vi "Demo Multitouch.vi"(8 "error in (no error)":errorcluster) -> (0 "error out":errorcluster)   [LabVIEW 2011]
uses:
  VIremote.llb/VIremoteEvent.ctl
  VIremote.llb/VIremoteFunction.ctl
  <vilib>/Utility/miscctls.llb/LVPointTypeDef.ctl
  <vilib>/Utility/miscctls.llb/LVPositionTypeDef.ctl
  VIremote.llb/VIremoteTouchPhase.ctl
panel:
  out "VIremoteEvent":T1=enum."Connection Closed"
  out "2D Picture":picture
  # "Touch with one finger to draw.\nTouch with two fingers to draw a line between them."
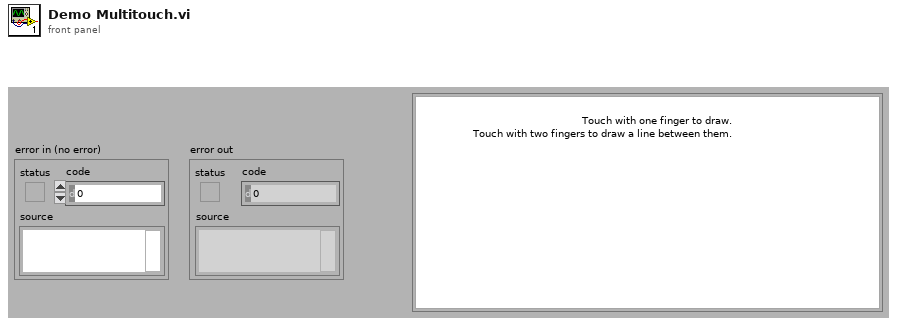
[diagram p1: front panel]
types:
  T1 = typedef "VIremoteEvent.ctl" = enum16{"No Event", "Connection Closed", "Navigate Back", "Enter Background", "Enter Foreground", "Portrait", "Portrait Upside Down", "Landscape Left", "Landscape Right"}
  T2 = typedef "LVPositionTypeDef.ctl" = cluster{"Left":i32, "Top":i32}
  T3 = typedef "LVPointTypeDef.ctl" = cluster{"Horizontal":i16, "Vertical":i16}
  T4 = typedef "VIremoteFunction.ctl" = enum16{"Do nothing", "Stop controller", "Close this connection", "Show info panel", "Set VI to control", "Set Accelerometer freq (Hz)", "Show Alert message", "Start Sound Input", "Stop Sound Input", "Set Volume (0-100)", "Set sound output Speaker", "Set sound output Receiver", "Play Sound", "Repeat Sound", "Stop Sound", "Pause Sound", "Resume Sound", "Set panel width of caller (320 or 480)", "Set Panel Size to Portrait", "Set Panel Size to Landscape", "Set Panel Size as Current Orientation", "Allow all UI Orientations", "Send user notification", "Disable Scrolling", "Normal Scrolling", "Page Scrolling", "Set Scroll Offset", "Page Indicator Position"}
  T5 = cluster{"UIorientation":refnum<notifier>, "Accelerometer":refnum<notifier>, "Sound":refnum<notifier>, "SoundPlayBufferReady":refnum<notifier>, "BackgroundState":refnum<notifier>, "Touch":refnum<notifier>}
  T6 = typedef "VIremoteTouchPhase.ctl" = enum32{"Began", "Moved", "Stationary", "Ended", "Cancelled"}
  T7 = cluster{"Width":u16, "Style":enum32{"Solid", "Dash", "Dot", "DashDot", "DashDotDot"}}
  T8 = typedef "VIremoteTouch.ctl" = cluster{"# touches":i32, "Touch phase":T6, "X":dbl, "Y":dbl, "Tap count":i32, "Timestamp":dbl, "ID":u32}
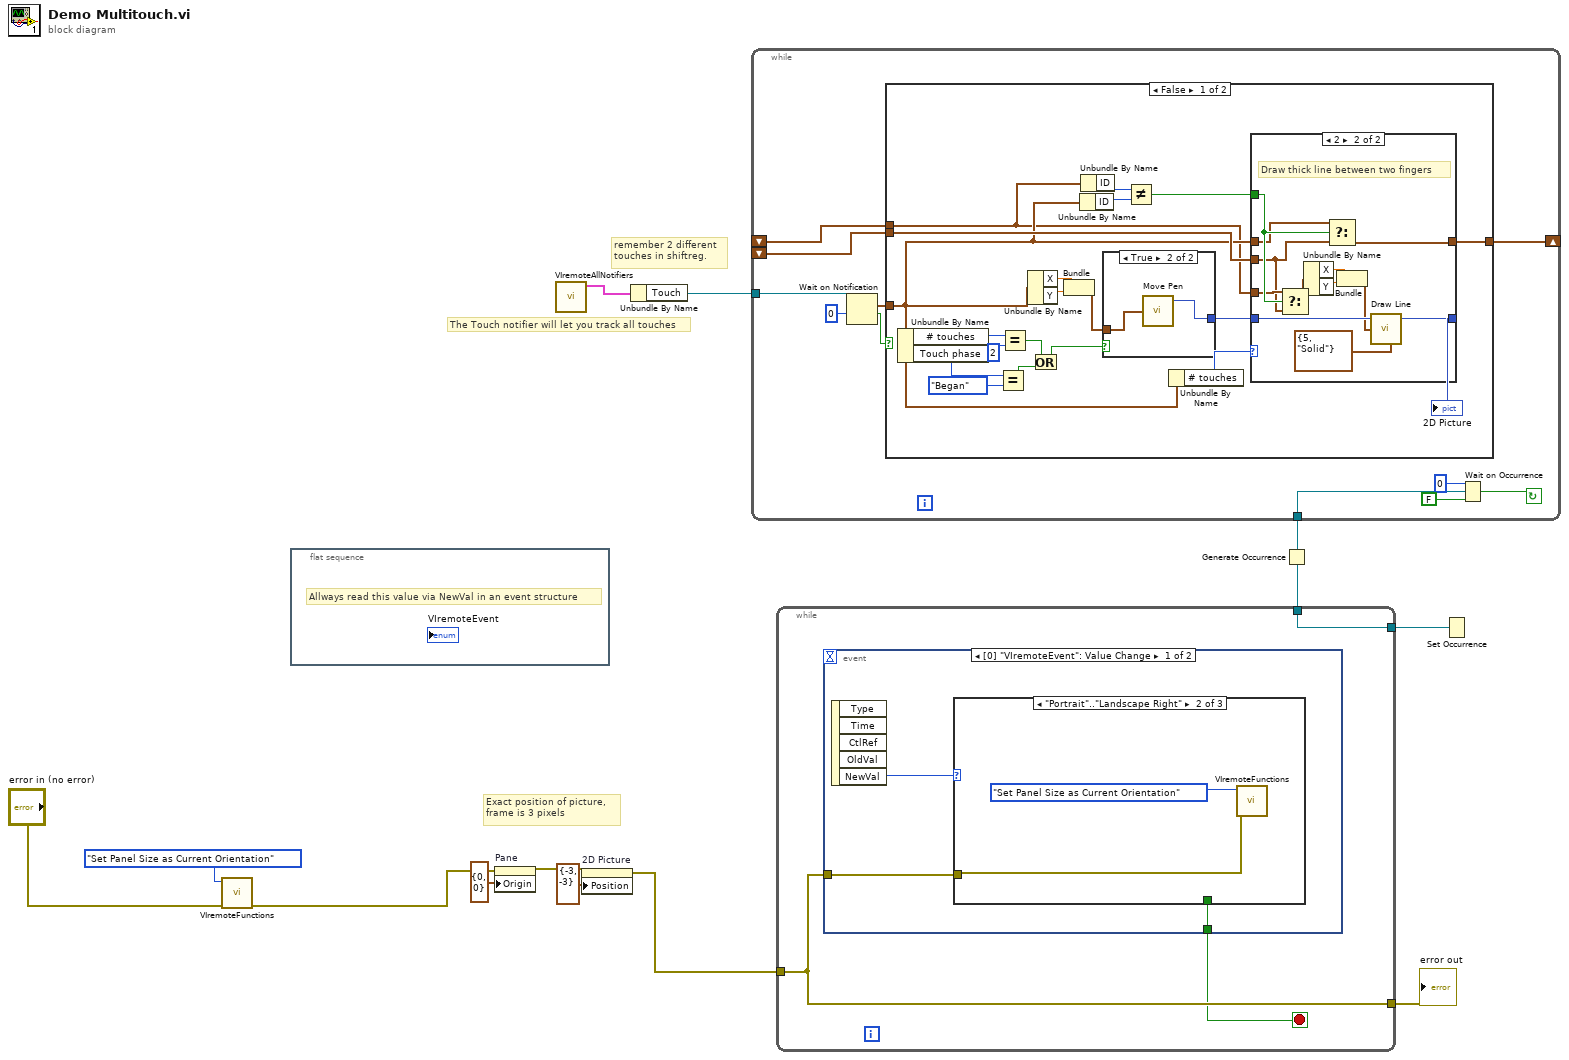
[diagram p0: block diagram]
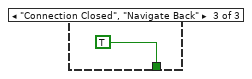
[diagram p3: hidden frame]
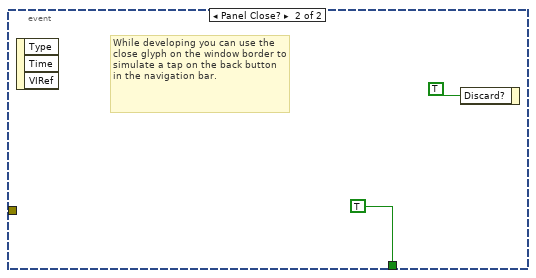
[diagram p4: hidden frame]
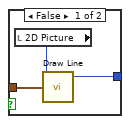
[diagram p6: hidden frame]
diagram:
  # "The Touch notifier will let you track all touches"
  # "Exact position of picture, \nframe is 3 pixels"
  # "remember 2 different\ntouches in shiftreg."
  n1 = call "VIremoteFunctions.vi"("error in (no error)"="error in (no error)", "Function"=VIremoteFunction."Set Panel Size as Current Orientation") -> ("error out"=w1:errorcluster)  [unwired: 4 in, 5 out]
  n2 = flat-sequence {
    frame #0 {
      # "Allways read this value via NewVal in an event structure"
    }
  }
  n3 = property on="Pane" class="Pane"(error in=w1, "Origin"=T3 {"Horizontal"=0, "Vertical"=0}) -> (error out=w6:errorcluster)  [unwired: 1 in, 1 out]
  n4 = call "VIremoteAllNotifiers.vi"() -> ("All Notifiers (unbundle by name)"=w11:T5)  [unwired: 1 in, 10 out]
  n5 = property on="2D Picture" class="Pict"(error in=w6, "Position"=T2 {"Left"=-3, "Top"=-3}) -> (error out=w5:errorcluster)  [unwired: 1 in, 1 out]
  n6 = Unbundle By Name(w11) -> ("Touch"=w10:refnum<notifier>)
  n7 = Generate Occurrence() -> (w3:refnum<k4>)
  n8 = while {
    tunnel: w10 -> [w23]
    shift-right: [w22] -> _
    shift-left: _ -> [w21]
    shift-left: _ -> [w20]
    tunnel: w3 -> [w16]
    stop <- w13 continue-if-true
    n9 = Wait on Notification(notifier=w23, timeout in ms (-1)=0) -> (notification=w19:T8, timed out?=w17:bool)  [unwired: 1 in, 3 out]
    n10 = case shown="False" w17 {
      tunnel: w19 -> [w25 _]
      tunnel: [w28 w63] -> w22
      tunnel: w21 -> [w24 _]
      tunnel: w20 -> [w26 w63]
      frame False {
        n11 = Unbundle By Name(w25) -> ("# touches"=w41:i32, "Touch phase"=w39:T6)
        n12 = Equal?(x=w39, y=VIremoteTouchPhase."Began") -> (x = y?=w33:bool)
        n13 = Equal?(x=w41, y=2) -> (x = y?=w32:bool)
        n14 = Unbundle By Name(w25) -> ("X"=w43:dbl, "Y"=w42:dbl)
        n15 = Or(x=w32, y=w33) -> (x .or. y?=w31:bool)
        n16 = Bundle("X"=w43, "Y"=w42) -> (w34:cluster{"X":dbl, "Y":dbl})  [unwired: 1 out]
        n17 = Unbundle By Name(w25) -> ("ID"=w29:u32)
        n18 = Unbundle By Name(w24) -> ("ID"=w30:u32)
        n19 = case shown="True" w31 {
          tunnel: w34 -> [w60 w61]
          tunnel: [w59 w62] -> w36
          frame False {
            n20 = local read "2D Picture"() -> (w58:picture)
            n21 = call <vilib>:"Draw Line.vi"("picture"=w58, "end point"=w60) -> ("new picture"=w59:picture)  [unwired: 3 in, 4 out]
          }
          frame True {
            n22 = call <vilib>:"Move Pen.vi"("new position"=w61) -> ("new picture"=w62:picture)  [unwired: 2 in, 2 out]
          }
        }
        n23 = Not Equal?(x=w30, y=w29) -> (x != y?=w27:bool)
        n24 = Unbundle By Name(w25) -> ("# touches"=w37:i32)
        n25 = case shown="2" w37 {
          tunnel: w36 -> [w45 w57]
          tunnel: [w45 w56] -> w35
          tunnel: [w44 w49] -> w28
          tunnel: w27 -> [_ w51]
          tunnel: w26 -> [_ w47]
          tunnel: w25 -> [w44 w50]
          tunnel: w24 -> [_ w48]
          frame 1, Default {
          }
          frame 2 {
            # "Draw thick line between two fingers"
            n26 = Select(t=w48, s=w51, f=w47) -> (s? t:f=w52:T8)
            n27 = Unbundle By Name(w52) -> ("X"=w54:dbl, "Y"=w55:dbl)
            n28 = Select(t=w50, s=w51, f=w47) -> (s? t:f=w49:T8)
            n29 = Bundle("X"=w54, "Y"=w55) -> (w53:cluster{"X":dbl, "Y":dbl})  [unwired: 1 out]
            n30 = call <vilib>:"Draw Line.vi"("picture"=w57, "end point"=w53, "pen"=T7 {"Width"=5, "Style"=enum."Solid"}) -> ("new picture"=w56:picture)  [unwired: 2 in, 4 out]
          }
        }
        "2D Picture" <- w35
      }
      frame True {
      }
    }
    n31 = Wait on Occurrence(1:FALSE ("ignore previous (T)"), 2:w16, 3:0 ("ms timeout (-1)")) -> (0:w13:bool)
  }
  n32 = while {
    tunnel: w5 -> [w66]
    tunnel: [w66] -> w2
    tunnel: [w64] -> w4
    tunnel: w3 -> [w64]
    stop <- w65 stop-if-true
    n33 = event shown="[0] \"VIremoteEvent\": Value Change" {
      selector: _ -> [_ _]
      dyn-events: _ -> [_ _]
      timeout: _ -> [_ _]
      tunnel: w66 -> [w69 _]
      tunnel: [w67 TRUE ("Discard?")] -> w65
      event Value Change {
        n34 = event-data() -> ("NewVal"=w68:T1)  [unwired: 5 out]
        n35 = case shown="\"Portrait\"..\"Landscape Right\"" w68 {
          tunnel: w69 -> [_ w71 _]
          tunnel: [_ _ TRUE] -> w67
          frame "No Event", Default {
          }
          frame "Portrait".."Landscape Right" {
            n36 = call "VIremoteFunctions.vi"("error in (no error)"=w71, "Function"=VIremoteFunction."Set Panel Size as Current Orientation") -> ()  [unwired: 4 in, 6 out]
          }
          frame "Connection Closed", "Navigate Back" {
          }
        }
      }
      event Panel Close? {
        # "While developing you can use the close glyph on the window border to simulate a tap on the back button in the navigation bar."
        n37 = event-data() -> ()  [unwired: 4 out]
        n38 = event-data("Discard?"=TRUE) -> ()  [unwired: 1 in, 1 out]
      }
    }
  }
  "error out" <- w2
  n39 = Set Occurrence(w4) -> ()
